vi "Teleop_Calc_dT.vi"(11 "Teleop Local Data in":T1) -> (3 "Teleop Local Data out":T1)   [LabVIEW 2016]
uses:
  Typedefs/typedef_cluster_Teleop Local Data.ctl
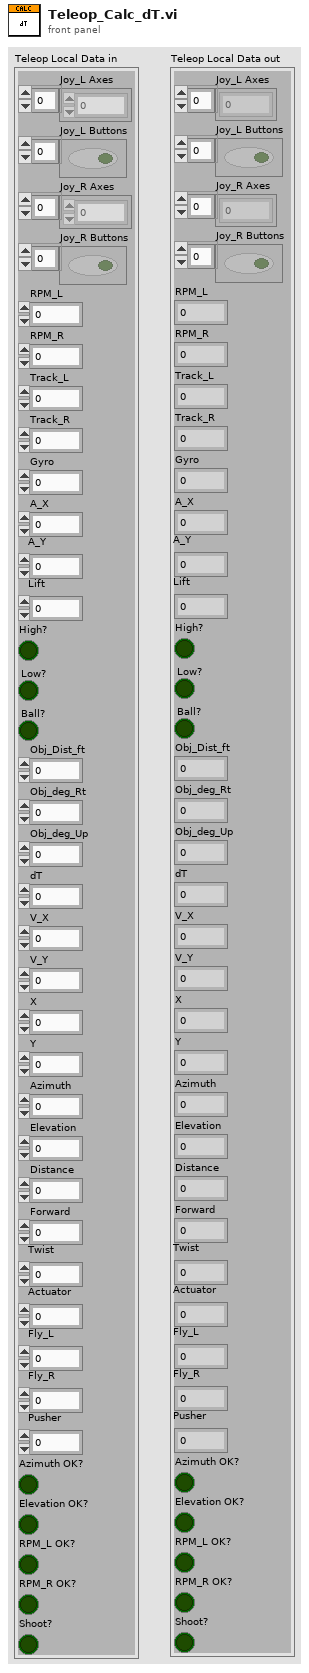
[diagram p1: front panel]
types:
  T1 = typedef "typedef_cluster_Teleop Local Data.ctl" = cluster{"Joy_L Axes":dbl[], "Joy_L Buttons":bool[], "Joy_R Axes":dbl[], "Joy_R Buttons":bool[], "RPM_L":dbl, "RPM_R":dbl, "Track_L":dbl, "Track_R":dbl, "Gyro":dbl, "A_X":dbl, "A_Y":dbl, "Lift":dbl, "High?":bool, "Low?":bool, "Ball?":bool, "Obj_Dist_ft":dbl, "Obj_deg_Rt":dbl, "Obj_deg_Up":dbl, "dT":dbl, "V_X":dbl, "V_Y":dbl, "X":dbl, "Y":dbl, "Azimuth":dbl, "Elevation":dbl, "Distance":dbl, "Forward":dbl, "Twist":dbl, "Actuator":dbl, "Fly_L":dbl, "Fly_R":dbl, "Pusher":dbl, "Azimuth OK?":bool, "Elevation OK?":bool, "RPM_L OK?":bool, "RPM_R OK?":bool, "Shoot?":bool}
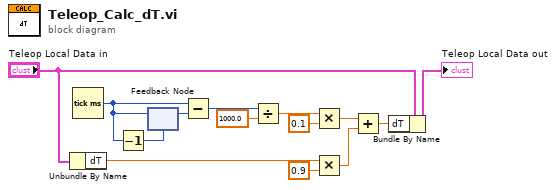
[diagram p0: block diagram]
diagram:
  n1 = Unbundle By Name("Teleop Local Data in") -> ("dT"=w7:dbl)
  n2 = Tick Count (ms)() -> (millisecond timer value=w11:u32)
  n3 = Decrement(x=w11) -> (x-1=w9:u32)
  n4 = feedback #1(w9) -> (w10:u32)
  n5 = feedback-in #1(w11) -> ()
  n6 = Subtract(x=w11, y=w10) -> (x-y=w12:u32)
  n7 = Divide(x=w12, y=1000.0) -> (x/y=w4:dbl)
  n8 = Multiply(x=w4, y=0.1) -> (x*y=w6:dbl)
  n9 = Multiply(x=w7, y=0.9) -> (x*y=w5:dbl)
  n10 = Add(x=w6, y=w5) -> (x+y=w3:dbl)
  n11 = Bundle By Name(cluster="Teleop Local Data in", "dT"=w3) -> (→"Teleop Local Data out":T1)
